vi "Resume.vi"(8 "error in (no error)":errorcluster, 11 "Execution in":refnum<class "Execution.lvclass">) -> (0 "error out":errorcluster, 3 "Execution out":refnum<class "Execution.lvclass">)   [LabVIEW 2020, in "TSnax.lvlib" / "Execution.lvclass"]
uses:
  Execution.lvclass
  Execution.lvclass/Execution.ctl
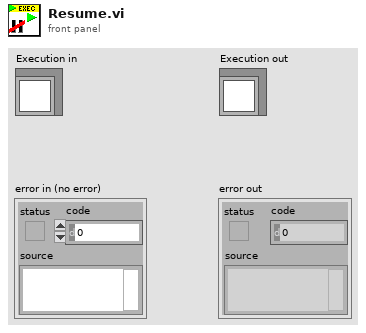
[diagram p1: front panel]
types:
  T1 = typedef "TSnax.lvlib/Execution.lvclass/Ref Data.ctl" = cluster{"Parameters":refnum<class "PropertyObject.lvclass">, "Client Sequence":refnum<class "SequenceFile.lvclass">, "Process Model":refnum<class "SequenceFile.lvclass">, "Entry Sequence":string, "Execution":refnum<k7>, "Report":refnum<class "Report.lvclass">, "Options":T2}
  T2 = typedef "TSnax.lvlib/Execution.lvclass/Execution Options.ctl" = cluster{"Use Default Model":bool, "Release Related Sessions":bool}
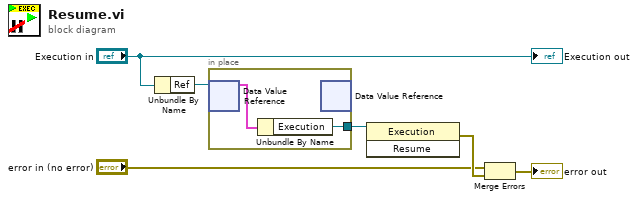
[diagram p0: block diagram]
diagram:
  n1 = Unbundle By Name("Execution in") -> ("Ref"=w6:refnum<data-value>)
  n2 = in-place {
    in-place-border: [w7] -> w5
    n3 = in-place-dvr #1(w6) -> (w8:T1)  [unwired: 1 out]
    n4 = Unbundle By Name(w8) -> ("Execution"=w7:refnum<k7>)
    n5 = in-place-dvr #1() -> ()  [unwired: 1 in, 2 out]
  }
  n6 = invoke class="Execution" method="Resume"(reference=w5) -> (error out=w4:errorcluster)  [unwired: 2 in, 2 out]
  n7 = Merge Errors("error in (no error)", w4) -> (→"error out":errorcluster)
  "Execution out" <- "Execution in"
